vi "DNatt Simple Solver.vi"(6 "Data":variant, 11 "Previous Guess Result":string) -> (3 "New Guess":string)   [LabVIEW 2020]
uses:
  <vilib>/numeric/Random Number (Range) U64.vi
  Libraries/Wordle Engine/Delete String Array Element.vi/fe6ff793-1998-4283-98d7-6c1f135b3a18.vi
  <vilib>/numeric/sub_Random U32.vi
  Libraries/Wordle Engine/Delete String Array Element.vi/fe6ff793-1998-4283-98d7-6c1f135b3a18.vi/d4db2432-cc9c-482c-8957-dac855435ef6.vi
  Libraries/Wordle Engine/Delete String Array Element.vi/fe6ff793-1998-4283-98d7-6c1f135b3a18.vi/86fbf154-bd7b-49a2-8ab2-a837b2a95f24.vi
  Libraries/Wordle Engine/Delete String Array Element.vi/fe6ff793-1998-4283-98d7-6c1f135b3a18.vi/3b95b01e-1ec2-4565-bcd9-7606a5281010.vi
  Libraries/Wordle Engine/Delete String Array Element.vi/fe6ff793-1998-4283-98d7-6c1f135b3a18.vi/96a08935-737a-44b2-979c-a81d56408f7e.vi
  Libraries/Wordle Engine/Delete String Array Element.vi/fe6ff793-1998-4283-98d7-6c1f135b3a18.vi/d4db2432-cc9c-482c-8957-dac855435ef6.vi/6eaecd13-6e48-4772-a921-b51ebdf84d88.vi
  Libraries/Wordle Engine/Delete String Array Element.vi/fe6ff793-1998-4283-98d7-6c1f135b3a18.vi/d4db2432-cc9c-482c-8957-dac855435ef6.vi/d2d5f2b7-06f4-47f6-971c-049c3fdbb653.vi
  Libraries/Wordle Engine/Delete String Array Element.vi/fe6ff793-1998-4283-98d7-6c1f135b3a18.vi/3b95b01e-1ec2-4565-bcd9-7606a5281010.vi/6eaecd13-6e48-4772-a921-b51ebdf84d88.vi
  Libraries/Wordle Engine/Delete String Array Element.vi/fe6ff793-1998-4283-98d7-6c1f135b3a18.vi/3b95b01e-1ec2-4565-bcd9-7606a5281010.vi/d2d5f2b7-06f4-47f6-971c-049c3fdbb653.vi
  Libraries/Wordle Engine/Delete String Array Element.vi/fe6ff793-1998-4283-98d7-6c1f135b3a18.vi/96a08935-737a-44b2-979c-a81d56408f7e.vi/6eaecd13-6e48-4772-a921-b51ebdf84d88.vi
  Libraries/Wordle Engine/Delete String Array Element.vi/fe6ff793-1998-4283-98d7-6c1f135b3a18.vi/96a08935-737a-44b2-979c-a81d56408f7e.vi/d2d5f2b7-06f4-47f6-971c-049c3fdbb653.vi
  <vilib>/Comparison/Less/Less Functor/Less Functor.lvclass
  Libraries/Wordle Engine/Wordle Engine.lvlib
panel:
  # "Note: Do not change the connector pane of this VI."
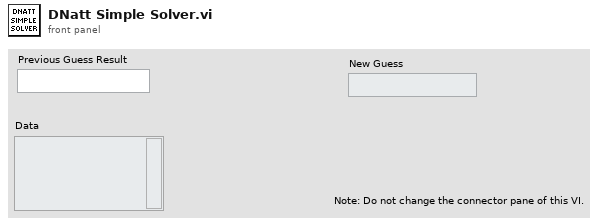
[diagram p1: front panel]
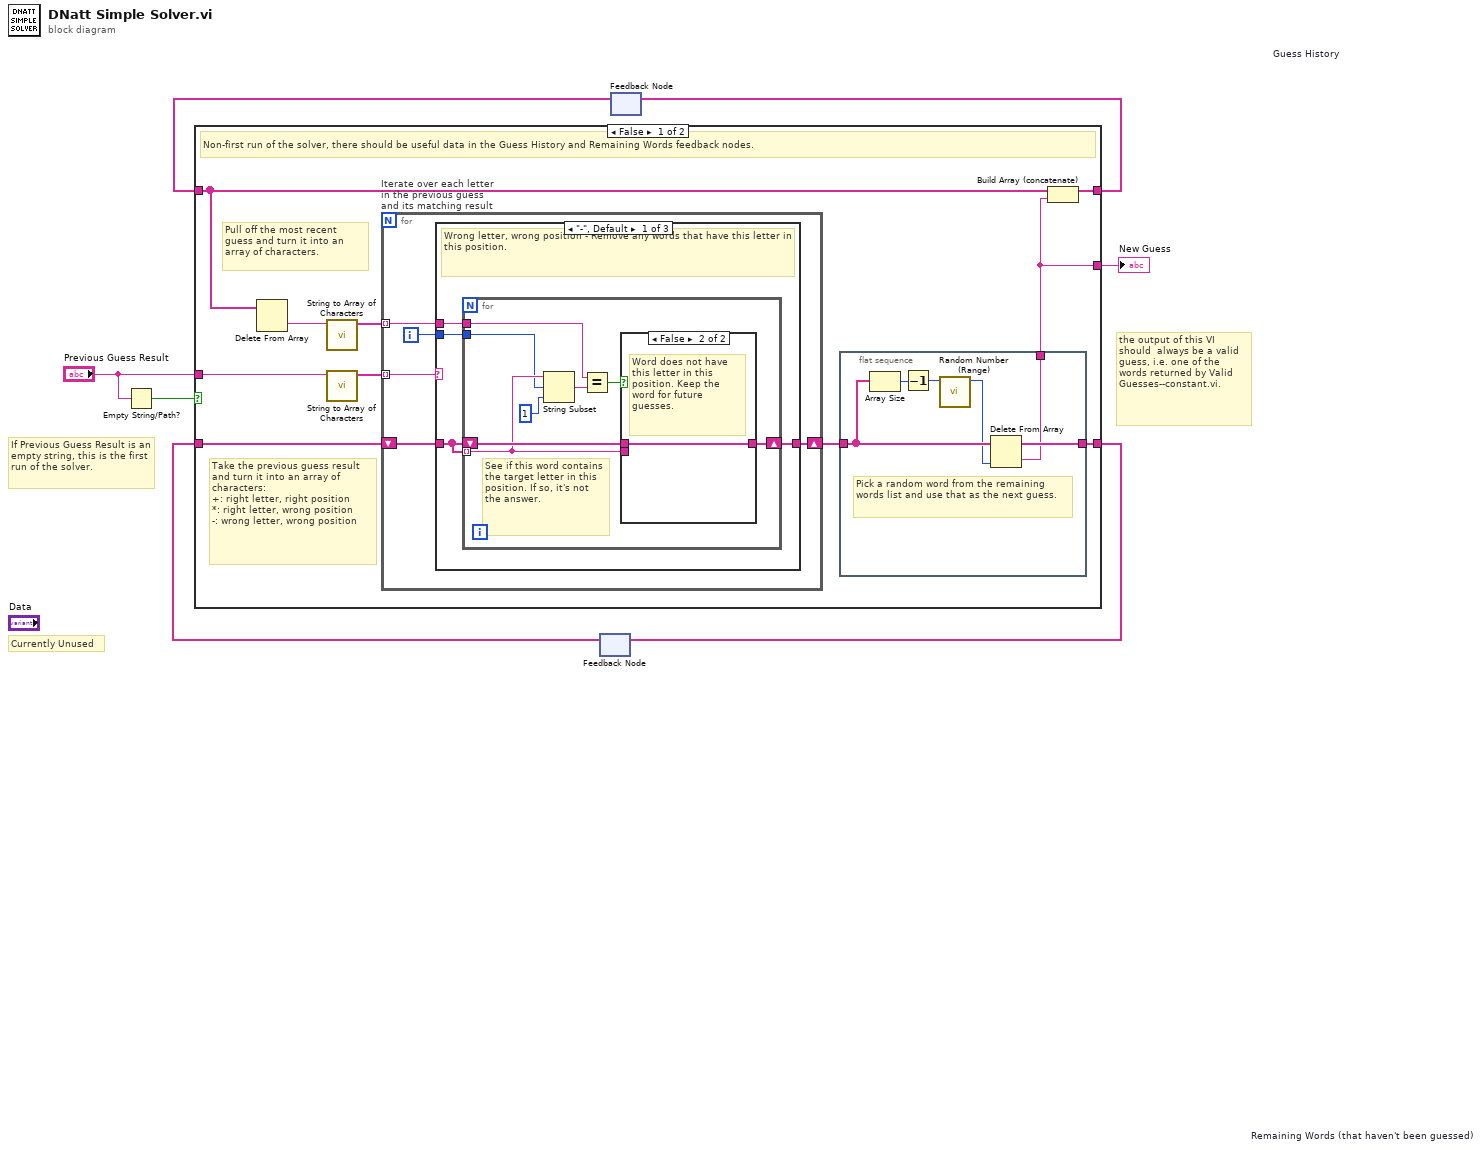
[diagram p0: block diagram]
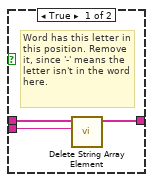
[diagram p2: hidden frame]
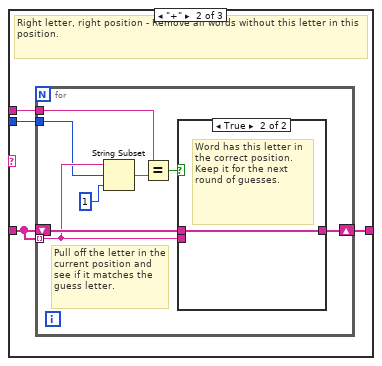
[diagram p3: hidden frame]
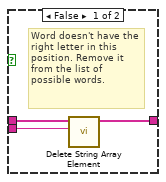
[diagram p4: hidden frame]
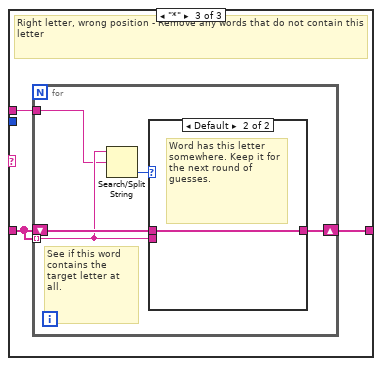
[diagram p5: hidden frame]
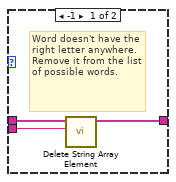
[diagram p6: hidden frame]
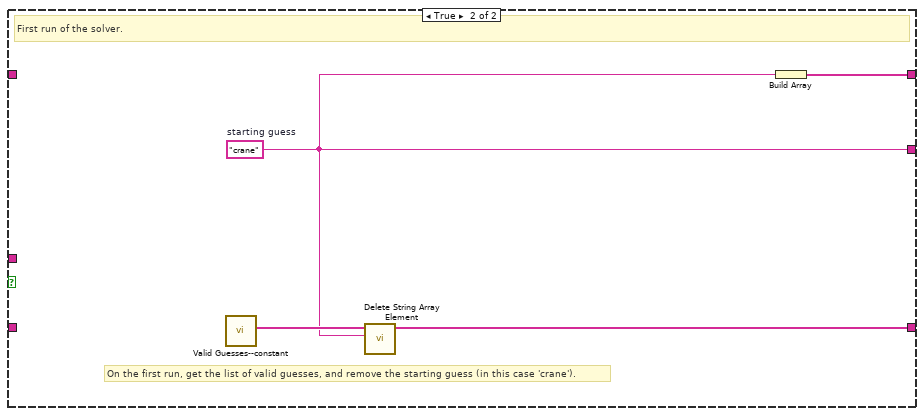
[diagram p7: hidden frame]
diagram:
  # "the output of this VI should  always be a valid guess, i.e. one of the words returned by Valid Guesses--constant.vi."
  # "If Previous Guess Result is an empty string, this is the first run of the solver."
  # "Currently Unused"
  n1 = Empty String/Path?(string/path="Previous Guess Result") -> (empty?=w1:bool)
  n2 = feedback #1 "Remaining Words (that haven't been guessed)"() -> (w3:string[])  [unwired: 1 in]
  n3 = feedback #2 "Guess History"() -> (w5:string[])  [unwired: 1 in]
  n4 = case shown="False" w1 {
    tunnel: [w9 w73] -> w7
    tunnel: [w16 w76] -> w6
    tunnel: w5 -> [w17 _]
    tunnel: "Previous Guess Result" -> [w14 _]
    tunnel: [w10 w74] -> w4
    tunnel: w3 -> [w8 _]
    frame False {
      # "Take the previous guess result and turn it into an array of characters:\n+: right letter, right position\n*: right letter, wrong position\n-: wrong letter, wrong position"
      # "Pull off the most recent guess and turn it into an array of characters."
      # "Non-first run of the solver, there should be useful data in the Guess History and Remaining Words feedback nodes."
      n5 = Delete From Array(array=w17) -> (deleted portion=w15:string)  [unwired: 2 in, 1 out]
      n6 = call "String to Array of Characters.vi"("String"=w15) -> ("Array of Characters"=w12:string[])  [unwired: 10 in]
      n7 = call "String to Array of Characters.vi"("String"=w14) -> ("Array of Characters"=w13:string[])  [unwired: 10 in]
      n8 = for "Iterate over each letter in the previous guess and its matching result" {
        tunnel: w13 -> [w28] mode=indexing
        tunnel: w12 -> [w27] mode=indexing
        shift-right: [w25] -> w11
        shift-left: w8 -> [w26]
        i -> [w24]
        n9 = case shown="\"-\", Default" w28 {
          tunnel: w27 -> [w31 w47 w62]
          tunnel: w26 -> [w30 w46 w61]
          tunnel: [w32 w48 w63] -> w25
          tunnel: w24 -> [w29 w45 _]
          frame "-", Default {
            # "Wrong letter, wrong position - Remove any words that have this letter in this position."
            n10 = for {
              tunnel: w30 -> [w37] mode=indexing
              shift-right: [w39] -> w32
              shift-left: w30 -> [w40]
              tunnel: w31 -> [w34]
              tunnel: w29 -> [w36]
              # "See if this word contains the target letter in this position. If so, it's not the answer."
              n11 = String Subset(string=w37, offset (0)=w36, length (rest)=1 ("length (rest)")) -> (substring=w35:string)
              n12 = Equal?(x=w34, y=w35) -> (x = y?=w33:bool)
              n13 = case shown="False" w33 {
                tunnel: w40 -> [w42 w44]
                tunnel: [w43 w44] -> w39
                tunnel: w37 -> [w41 _]
                frame True {
                  # "Word has this letter in this position. Remove it, since '-' means the letter isn't in the word here."
                  n14 = call "Delete String Array Element.vi"("Element to Delete"=w41, "Array in"=w42) -> ("Array out"=w43:string[])  [unwired: 8 in, 1 out]
                }
                frame False {
                  # "Word does not have this letter in this position. Keep the word for future guesses."
                }
              }
            }
          }
          frame "+" {
            # "Right letter, right position - Remove all words without this letter in this position."
            n15 = for {
              tunnel: w46 -> [w51] mode=indexing
              shift-right: [w55] -> w48
              shift-left: w46 -> [w56]
              tunnel: w47 -> [w49]
              tunnel: w45 -> [w50]
              # "Pull off the letter in the current position and see if it matches the guess letter."
              n16 = String Subset(string=w51, offset (0)=w50, length (rest)=1 ("length (rest)")) -> (substring=w53:string)
              n17 = Equal?(x=w49, y=w53) -> (x = y?=w52:bool)
              n18 = case shown="True" w52 {
                tunnel: w56 -> [w59 w60]
                tunnel: [w58 w60] -> w55
                tunnel: w51 -> [w57 _]
                frame False {
                  # "Word doesn't have the right letter in this position. Remove it from the list of possible words."
                  n19 = call "Delete String Array Element.vi"("Element to Delete"=w57, "Array in"=w59) -> ("Array out"=w58:string[])  [unwired: 8 in, 1 out]
                }
                frame True {
                  # "Word has this letter in the correct position. Keep it for the next round of guesses."
                }
              }
            }
          }
          frame "*" {
            # "Right letter, wrong position - Remove any words that do not contain this letter"
            n20 = for {
              tunnel: w61 -> [w66] mode=indexing
              shift-right: [w67] -> w63
              shift-left: w61 -> [w68]
              tunnel: w62 -> [w64]
              # "See if this word contains the target letter at all."
              n21 = Search/Split String(string=w66, search string/char (-)=w64) -> (offset of match=w65:i32)  [unwired: 1 in, 2 out]
              n22 = case shown="Default" w65 {
                tunnel: w68 -> [w71 w72]
                tunnel: [w70 w72] -> w67
                tunnel: w66 -> [w69 _]
                frame -1 {
                  # "Word doesn't have the right letter anywhere. Remove it from the list of possible words."
                  n23 = call "Delete String Array Element.vi"("Element to Delete"=w69, "Array in"=w71) -> ("Array out"=w70:string[])  [unwired: 8 in, 1 out]
                }
                frame Default {
                  # "Word has this letter somewhere. Keep it for the next round of guesses."
                }
              }
            }
          }
        }
      }
      n24 = flat-sequence {
        tunnel: w11 -> [w22]
        tunnel: [w21] -> w10
        tunnel: [w19] -> w9
        frame #0 {
          # "Pick a random word from the remaining words list and use that as the next guess."
          n25 = Array Size(array=w22) -> (size(s)=w23:i32)
          n26 = Decrement(x=w23) -> (x-1=w18:i32)
          n27 = call-poly <vilib>:"Random Number (Range).vi"("upper bound (100)"=w18) -> ("number"=w20:u64)  [unwired: 10 in]
          n28 = Delete From Array(array=w22, index=w20) -> (deleted portion=w19:string, array with subset deleted=w21:string[])  [unwired: 1 in]
        }
      }
      n29 = Build Array (concatenate)(w17, w9) -> (w16:string[])
    }
    frame True {
      w73 = "crane"  # starting guess
      # "On the first run, get the list of valid guesses, and remove the starting guess (in this case 'crane')."
      # "First run of the solver."
      n30 = call "Valid Guesses--constant.vi"() -> ("Valid Guesses (array)"=w75:string[])  [unwired: 10 in, 1 out]
      n31 = call "Delete String Array Element.vi"("Element to Delete"=w73, "Array in"=w75) -> ("Array out"=w74:string[])  [unwired: 8 in, 1 out]
      n32 = Build Array(w73) -> (w76:string[])
    }
  }
  "New Guess" <- w7
  n33 = feedback-in #1(w4) -> ()
  n34 = feedback-in #2(w6) -> ()
